vi "Initialize Database.vi"(8 "error in (no error)":errorcluster, 10 "Baud Rate":u32, 11 "Addon Name":string) -> (0 "error out":errorcluster, 2 "Cluster":refnum<k21>, 3 "XNET Database":refnum<k21>)   [LabVIEW 2015, in "Diagnostics Addon Engine.lvlib"]
uses:
  Diagnostics Addon Engine.lvlib
  Shared/CAN Cluster.ctl
  <vilib>/xnet/xnet.llb/XNET Database Open (Database).vi
  Shared/Diagnostics Addon Shared.lvlib
  <resource>/objmgr/xnet.rc
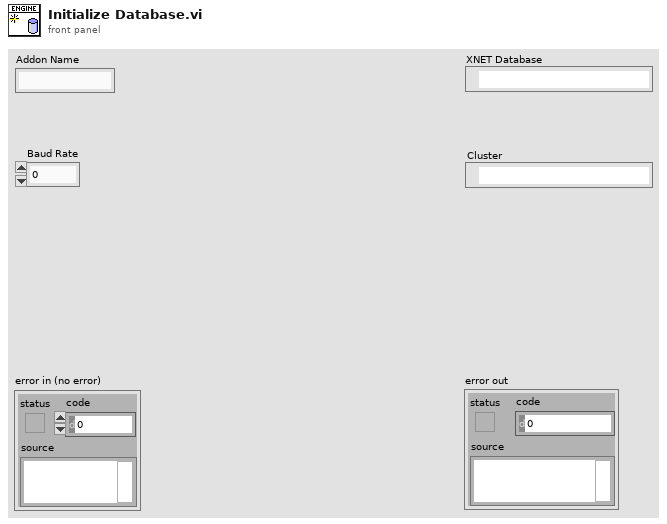
[diagram p1: front panel]
types:
  T1 = typedef "Diagnostics Addon Shared.lvlib/CAN Cluster.ctl" = cluster{"Baud Rate":u32, "Comment":string, "Name":string}
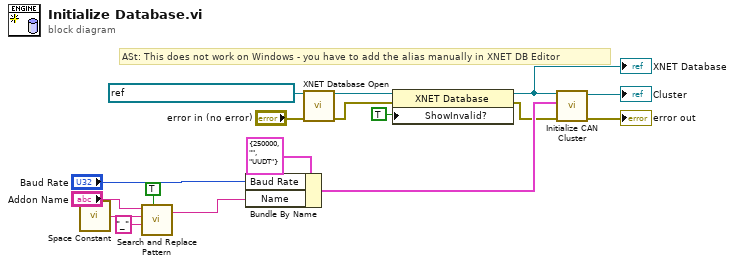
[diagram p0: block diagram]
diagram:
  # "ASt: This does not work on Windows - you have to add the alias manually in XNET DB Editor"
  n1 = call <vilib>:"Space Constant.vi"() -> ("String"=w10:string)
  n2 = call <vilib>:"Search and Replace Pattern.vi"("string"="Addon Name", "regular expression (\"\")"=w10, "replace string (\"\")"="_" ("replace string (\"\")"), "replace all? (F)"=TRUE) -> ("result string"=w8:string)  [unwired: 1 in, 1 out]
  n3 = Bundle By Name(cluster=T1 {"Baud Rate"=250000, "Comment"="", "Name"="UUDT"} ("CAN Cluster"), "Baud Rate"="Baud Rate", "Name"=w8) -> (w16:T1)
  n4 = call-poly <vilib>:"XNET Database Open.vi"("database in (:memory:)"=refnum<k21> "Diagnostics_Addon_Temp_DB", "error in (no error)"="error in (no error)") -> ("database out"=w2:refnum<k21>, "error out"=w6:errorcluster)  [unwired: 12 out]
  n5 = property class="XNET Database"(reference=w2, error in=w6, "ShowInvalid?"=TRUE ("Show Invalid From Open?")) -> (reference out=w7:refnum<k21>, error out=w5:errorcluster)
  "XNET Database" <- w7
  n6 = call "Initialize CAN Cluster.vi"("error in"=w5, "CAN Cluster"=w16, "database in"=w7) -> ("error out"=→"error out":errorcluster, "cluster out"=→"Cluster":refnum<k21>)  [unwired: 7 out]
